vi "Reply.vi"(8 "error in (no error)":errorcluster, 11 "Self-addressed Msg in":refnum<class "Self-addressed Msg.lvclass">) -> (0 "error out":errorcluster, 3 "Self-addressed Msg out":refnum<class "Self-addressed Msg.lvclass">)   [LabVIEW 2019, in "Self-addressed Msg.lvclass"]
uses:
  Self-addressed Msg.lvclass
  C:/Program Files/National Instruments/LabVIEW 2019/vi.lib/ActorFramework/Message/Message.lvclass
  Self-addressed Msg.lvclass/Self-addressed Msg.ctl
  <vilib>/ActorFramework/Message Enqueuer/Message Enqueuer.lvclass/Message Enqueuer.ctl
  <vilib>/ActorFramework/Message Priority Queue/Priority Enqueue.vi
  <vilib>/ActorFramework/Message Enqueuer/Message Enqueuer.lvclass
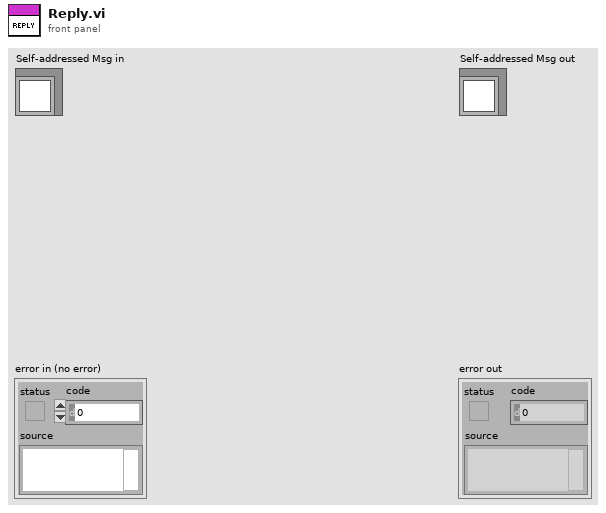
[diagram p1: front panel]
types:
  T1 = typedef "Actor Framework.lvlib/Message Enqueuer.lvclass/Message Priority.ctl" = enum16{"Low", "Normal", "High"}
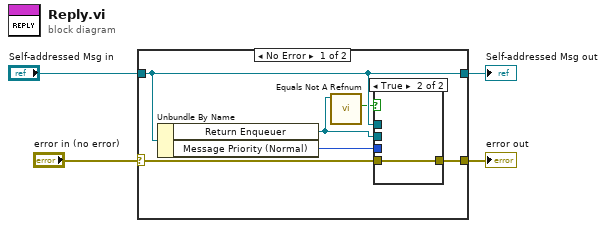
[diagram p0: block diagram]
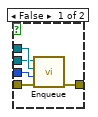
[diagram p2: hidden frame]
diagram:
  n1 = case shown="No Error" "error in (no error)" {
    selector: "error in (no error)" -> [w8 w18]
    tunnel: "Self-addressed Msg in" -> [w7 w17]
    tunnel: [w10 w18] -> w4
    tunnel: [w7 w17] -> w1
    frame No Error {
      n2 = Unbundle By Name(w7) -> ("Return Enqueuer"=w6:refnum<class "Message Enqueuer.lvclass">, "Message Priority (Normal)"=w9:T1)
      n3 = call <vilib>:"Equals Not A Refnum.vi"("Message Enqueuer"=w6) -> ("Not a refnum?"=w5:bool)  [unwired: 10 in]
      n4 = case shown="True" w5 {
        tunnel: [w15 w16] -> w10
        tunnel: w9 -> [w14 _]
        tunnel: w8 -> [w13 w16]
        tunnel: w7 -> [w12 _]
        tunnel: w6 -> [w11 _]
        frame False {
          n5 = call <vilib>:"Enqueue.vi"("error in (no error)"=w13, "Message Priority (Normal)"=w14, "Message"=w12, "Message Enqueuer in"=w11) -> ("error out"=w15:errorcluster)  [unwired: 6 in, 1 out]
        }
        frame True {
        }
      }
    }
    frame Error {
    }
  }
  "error out" <- w4
  "Self-addressed Msg out" <- w1
